vi "NI-Switch Initialization SubVI-Cancel.vi"(4 "Topology Name":string, 5 "Channels Array":string[](array[string]), 6 "Resource Name":string, 8 "error in (no error)":errorcluster, 9 "Custom XML":string, 11 "Device Item Ref in":T1 format="%.0x") -> (0 "error out":errorcluster, 3 "Device Item Ref out":T1 format="%.0x")   [LabVIEW 2010, in "NI-Switch Relay Custom Device.lvlib"]
uses:
  NI-Switch Relay Custom Device.lvlib
  <vilib>/NI Veristand/Custom Device API/Custom Device Item Ref.ctl
  <vilib>/NI Veristand/Custom Device API/Custom Device API.lvlib
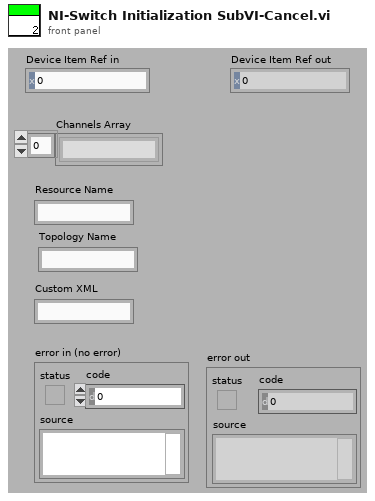
[diagram p1: front panel]
types:
  T1 = typedef "Custom Device API.lvlib/Custom Device Item Ref.ctl" = u64
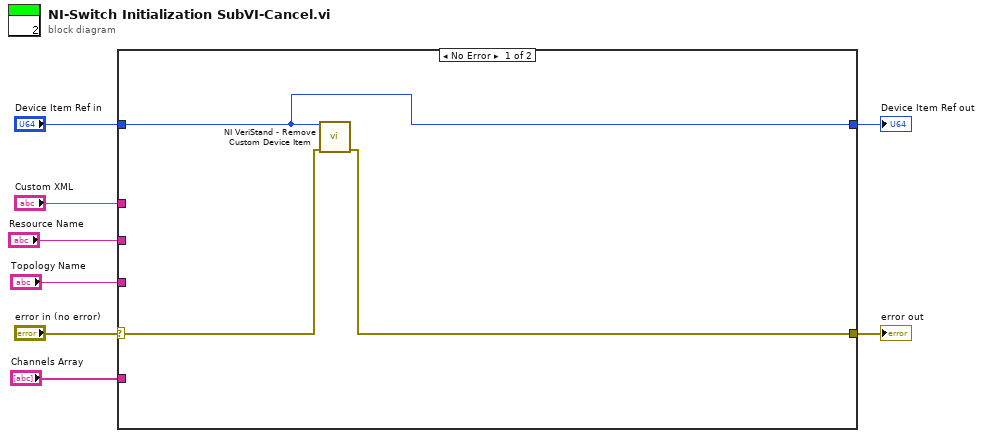
[diagram p0: block diagram]
diagram:
  n1 = case shown="No Error" "error in (no error)" {
    selector: "error in (no error)" -> [w11 w13]
    tunnel: [w10 w13] -> w4
    tunnel: [w9 w12] -> w6
    tunnel: "Device Item Ref in" -> [w9 w12]
    tunnel: "Custom XML" -> [_ _]
    tunnel: "Channels Array" -> [_ _]
    tunnel: "Resource Name" -> [_ _]
    tunnel: "Topology Name" -> [_ _]
    frame No Error {
      n2 = call <vilib>:"NI VeriStand - Remove Custom Device Item.vi"("error in (no error)"=w11, "Item Ref in"=w9) -> ("error out"=w10:errorcluster)  [unwired: 8 in, 1 out]
    }
    frame Error {
    }
  }
  "error out" <- w4
  "Device Item Ref out" <- w6
